vi "MergeRows.vi"(8 "error in (no error)":errorcluster, 9 "RowContent(Slave)":string[](array[string]), 10 "RowContent(Master)":string[](array[string]), 11 "List.lvclass":refnum<class "List.lvclass">) -> (0 "error out":errorcluster, 2 "NewContents":string[](array[string]), 3 "List.lvclass Out":refnum<class "List.lvclass">)   [LabVIEW 2015, in "List.lvclass"]
uses:
  List.lvclass
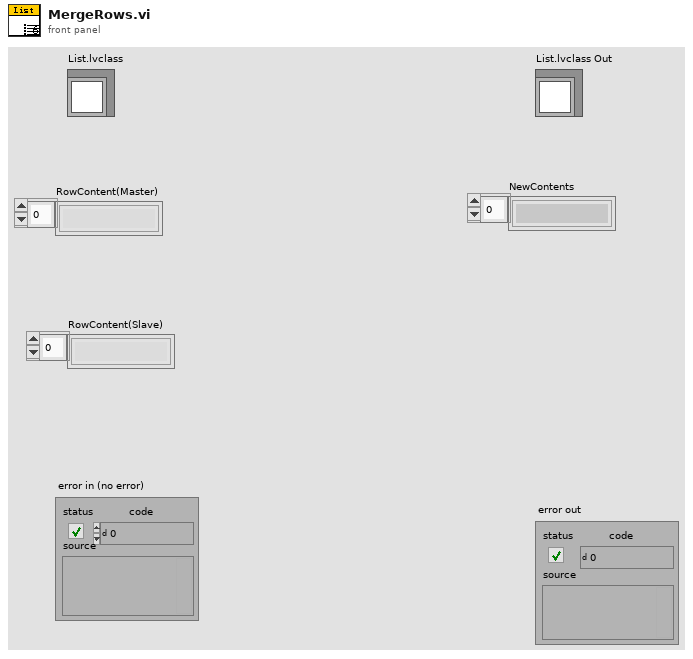
[diagram p1: front panel]
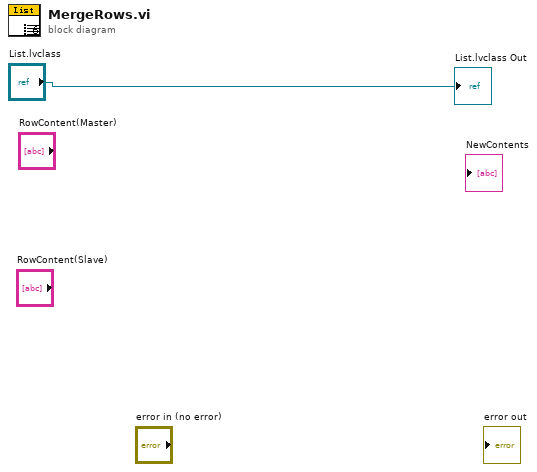
[diagram p0: block diagram]
diagram:
  "List.lvclass Out" <- "List.lvclass"
